vi "niusrprios Configure Signal.vi"   [LabVIEW 2015]
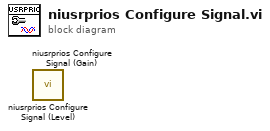
[diagram p0: block diagram]
diagram:
  n1 = call "niusrprios Configure Signal (Level).vi"() -> ()  [unwired: 9 in, 7 out]
  n2 = call "niusrprios Configure Signal (Gain).vi"() -> ()  [unwired: 9 in, 7 out]
